vi "Send.vi"(8 "error in (no error)":errorcluster, 10 "Message":refnum<class "MSG.lvclass">, 11 "Message Logger in":refnum<class "Message Logger.lvclass">) -> (0 "error out":errorcluster, 3 "Message Logger out":refnum<class "Message Logger.lvclass">)   [LabVIEW 2011, in "Messenging.lvlib" / "Message Logger.lvclass"]
uses:
  Message Logger.lvclass
  Parallel Process.lvclass
  MessageLoggerMessage/MessageLoggerMessage.lvclass
  Interprocess Messenger/TextVarientMessage/MSG.lvclass
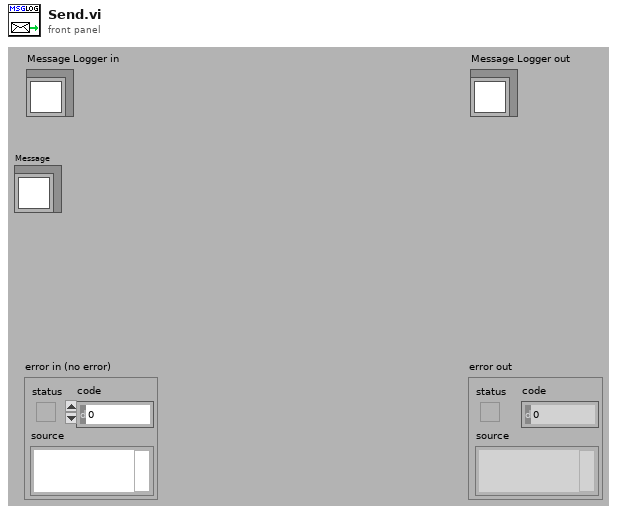
[diagram p1: front panel]
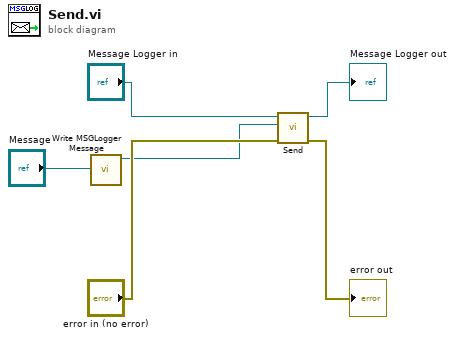
[diagram p0: block diagram]
diagram:
  n1 = call "Write MSGLogger Message.vi"("Message to Log"="Message") -> ("MessageLoggerMessage out"=w1:refnum<class "MessageLoggerMessage.lvclass">)  [unwired: 1 in, 9 out]
  n2 = call-parent "Send.vi"("error in (no error)"="error in (no error)", "Message"=w1, "Parallel Process in"="Message Logger in") -> ("error out"=→"error out":errorcluster, "Parallel Process out"=→"Message Logger out":refnum<class "Message Logger.lvclass">)  [unwired: 7 out]
